vi "not_ready.vi"(8 "error in (no error)":errorcluster, 11 "control references in":T1) -> (0 "error out":errorcluster, 3 "control references out":T1)   [LabVIEW 2010]
uses:
  type_definitions/clusters/controls_refs.ctl
  type_definitions/enumerations/main_control_types.ctl
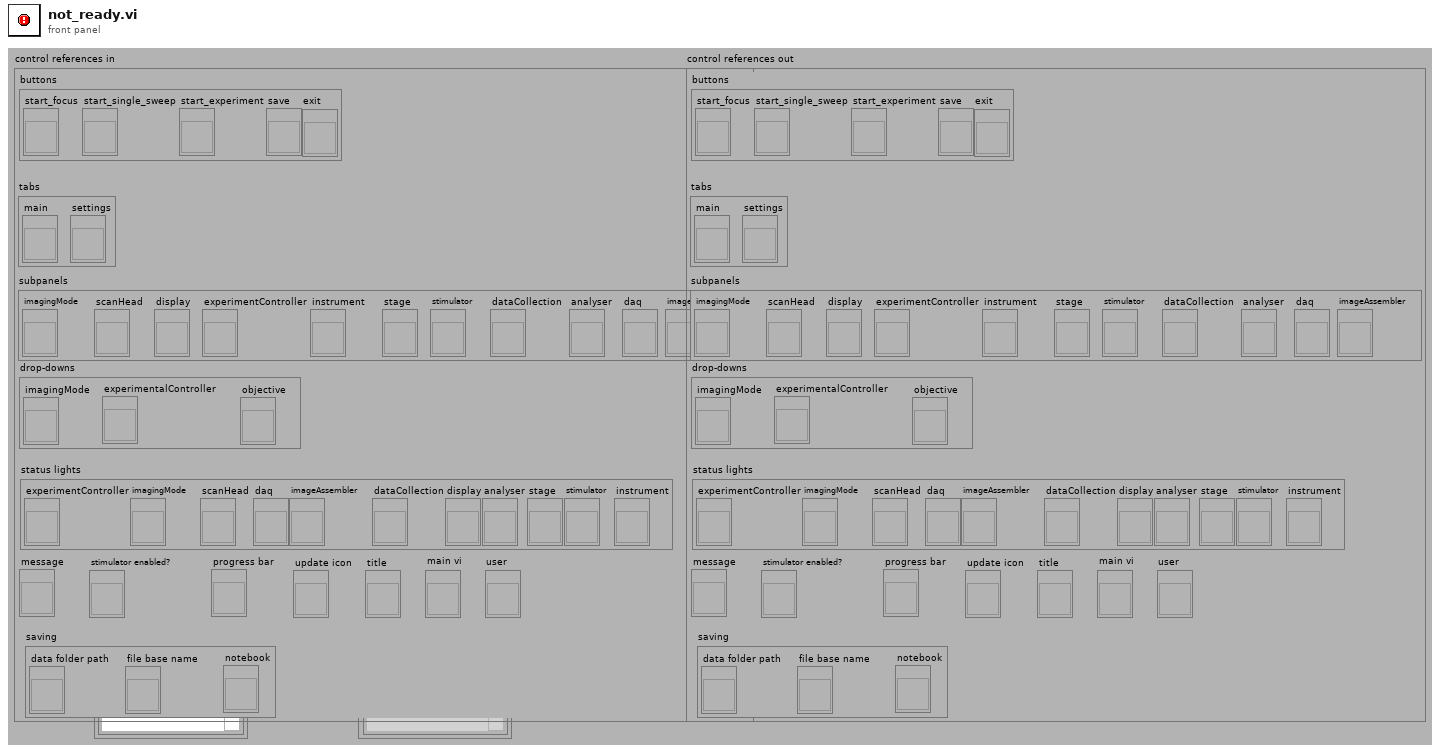
[diagram p1: front panel]
types:
  T1 = typedef "controls_refs.ctl" = cluster{"buttons":cluster{"start_focus":refnum<vi>, "start_single_sweep":refnum<vi>, "start_experiment":refnum<vi>, "save":refnum<vi>, "exit":refnum<vi>}, "tabs":cluster{"main":refnum<vi>, "settings":refnum<vi>}, "subpanels":cluster{"imagingMode":refnum<vi>, "scanHead":refnum<vi>, "display":refnum<vi>, "experimentController":refnum<vi>, "instrument":refnum<vi>, "stage":refnum<vi>, "stimulator":refnum<vi>, "dataCollection":refnum<vi>, "analyser":refnum<vi>, "daq":refnum<vi>, "imageAssembler":refnum<vi>}, "drop-downs":cluster{"imagingMode":refnum<vi>, "experimentalController":refnum<vi>, "objective":refnum<vi>}, "status lights":cluster{"experimentController":refnum<vi>, "imagingMode":refnum<vi>, "scanHead":refnum<vi>, "daq":refnum<vi>, "imageAssembler":refnum<vi>, "dataCollection":refnum<vi>, "display":refnum<vi>, "analyser":refnum<vi>, "stage":refnum<vi>, "stimulator":refnum<vi>, "instrument":refnum<vi>}, "message":refnum<vi>, "stimulator enabled?":refnum<vi>, "saving":cluster{"data folder path":refnum<vi>, "file base name":refnum<vi>, "notebook":refnum<vi>}, "progress bar":refnum<vi>, "update icon":refnum<vi>, "title":refnum<vi>, "main vi":refnum<vi>, "user":refnum<vi>}
  T2 = enum8{"Enabled", "Disabled", "Disabled and Grayed Out"}
  T3 = typedef "main_control_types.ctl" = enum16{"scan start button", "experimentController subpanel", "imagingMode subpanel", "scanHead subpanel", "dataCollection subpanel", "display subpanel", "analyser subpanel", "stimulator subpanel", "run mode drop-down", "imagingMode drop-down", "experimentController drop-down", "objective drop-down", "exit button"}
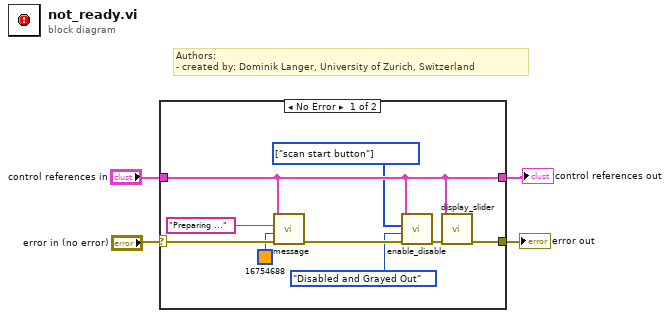
[diagram p0: block diagram]
diagram:
  # "Authors: \n- created by: Dominik Langer, University of Zurich, Switzerland"
  n1 = case shown="No Error" "error in (no error)" {
    selector: "error in (no error)" -> [w13 w15]
    tunnel: [w10 w15] -> w3
    tunnel: "control references in" -> [w7 w14]
    tunnel: [w7 w14] -> w1
    frame No Error {
      w6 = T3[] [enum."scan start button"] items=["scan start button", "experimentController subpanel", "imagingMode subpanel", "scanHead subpanel", "dataCollection subpanel", "display subpanel", "analyser subpanel", "stimulator subpanel", "run mode drop-down", "imagingMode drop-down", "experimentController drop-down", "objective drop-down", "exit button"] ("controls")
      n2 = call "message.vi"("error in (no error)"=w13, "BG slider"=u32 16754688, "text"="Preparing ...", "control references in"=w7) -> ("error out"=w9:errorcluster)  [unwired: 3 in, 4 out]
      n3 = call "enable_disable.vi"("error in (no error)"=w9, "state"=T2."Disabled and Grayed Out", "controls"=w6, "control references in"=w7) -> ("error out"=w8:errorcluster)  [unwired: 6 in, 1 out]
      n4 = call "display_slider.vi"("error in"=w8, "cluster refs in"=w7) -> ("error out"=w10:errorcluster)  [unwired: 9 in]
    }
    frame Error {
    }
  }
  "error out" <- w3
  "control references out" <- w1
